vi "test-discretization.vi"(8 "error in (no error)":errorcluster) -> (0 "error out":errorcluster, 3 "All Tests Passed":bool)   [LabVIEW 2019]
uses:
  <vilib>/Analysis/Matrix/Datatypes/RealMatrix.ctl
  <vilib>/Analysis/baseanly.llb/Real A x B.vi
  <vilib>/Rock Robotics/WPI/ThirdParty/JAS_Junk/TrajLib/MatBuilder_Create.vi
  <vilib>/Rock Robotics/WPI/ThirdParty/JAS_Junk/TrajLib/MatrixHelper_CoerceSize.vi
  <vilib>/Rock Robotics/WPI/ThirdParty/JAS_Junk/TrajLib/Matrix_Exp.vi
  <vilib>/Rock Robotics/WPI/ThirdParty/JAS_Junk/TrajLib/Matrix_AssignBlock.vi
  <vilib>/Rock Robotics/WPI/ThirdParty/JAS_Junk/TrajLib/Matrix_ExtractFrom.vi
  <vilib>/Analysis/7linalg.llb/Transpose Matrix.vi
  <vilib>/Analysis/7linalg.llb/Real Transpose Matrix.vi
  <vilib>/Rock Robotics/WPI/ThirdParty/JAS_Junk/TrajLib/Matrix_Ident.vi
  <vilib>/Analysis/7linalg.llb/Matrix Exp.vi
  <vilib>/Analysis/7linalg.llb/Real Matrix Exp.vi
  <vilib>/Analysis/Matrix/Numeric/Multiply/Multiply.vi
  <vilib>/Analysis/Matrix/Numeric/Multiply/Multiply - RM,R.vi
  <vilib>/Analysis/7linalg.llb/Create Special Matrix.vi
  <vilib>/Analysis/7linalg.llb/Create Special Real Matrix.vi
  <vilib>/Analysis/Matrix/Numeric/Add/Add - RM,RM.vi
  <vilib>/Analysis/Matrix/Comparison/Equal/Equal - RM,RM.vi
  <vilib>/Rock Robotics/WPI/ThirdParty/JAS_Junk/TrajLib/Trajectory_Library.lvlib
  <vilib>/Analysis/NI_AALBase.lvlib
  <vilib>/Analysis/Matrix/NI_Matrix.lvlib
panel:
  out "X1Discrete 11":T1
  out "DiscB  11":T1
  out "Passed 11":bool
  out "DiscA  11":T1
  out "Passed 10":bool
  out "DiscA  10":T1
  out "Passed 16":bool
  out "DiscR  16":T1
  out "A+B Should be":T1
  out "A + B":T1
  out "Test x passed":bool
  out "Test 3 passed":bool
  out "Test Passed 2":bool
  out "Test Passed 1":bool
  out "Test Passed 0":bool
  out "AQ Passed":bool
  out "AQ - DiscQ":T1
  out "AQ - DiscA":T1
  out "AB-Taylor-Passed":bool
  out "ABTaylor-DiscB":T1
  out "ABTaylor - DiscA":T1
  out "AB-passed":bool
  out "AB-DiscB":T1
  out "AB - DiscA":T1
  out "x1-Disc":T1
  out "DiscA Error":bool
  out "DiscA":T1
  out "Cost Mat":T1
  out "CoVar Mat":T1
  # "1.0,   0.0,    0.0\n\n0.0,     4.0,   0.0, ;\n\n0.0,     0.0,  9.0;"
  # "1.0,      0.0,      0.0, \n\n0.0,   1.0 / 4.0,   0.0, \n\n0.0,       0.0,      1.0 / 9.0,"
  # "VecBuilder.fill(\n          x0.get(0, 0) + 1.0 * x0.get(1, 0), \n          x0.get(1, 0));"
  # "2,\n1"
  # "x0.get(0, 0) + x0.get(1, 0) + 0.5 * u.get(0, 0), \n\nx0.get(0, 0) + u.get(0, 0))"
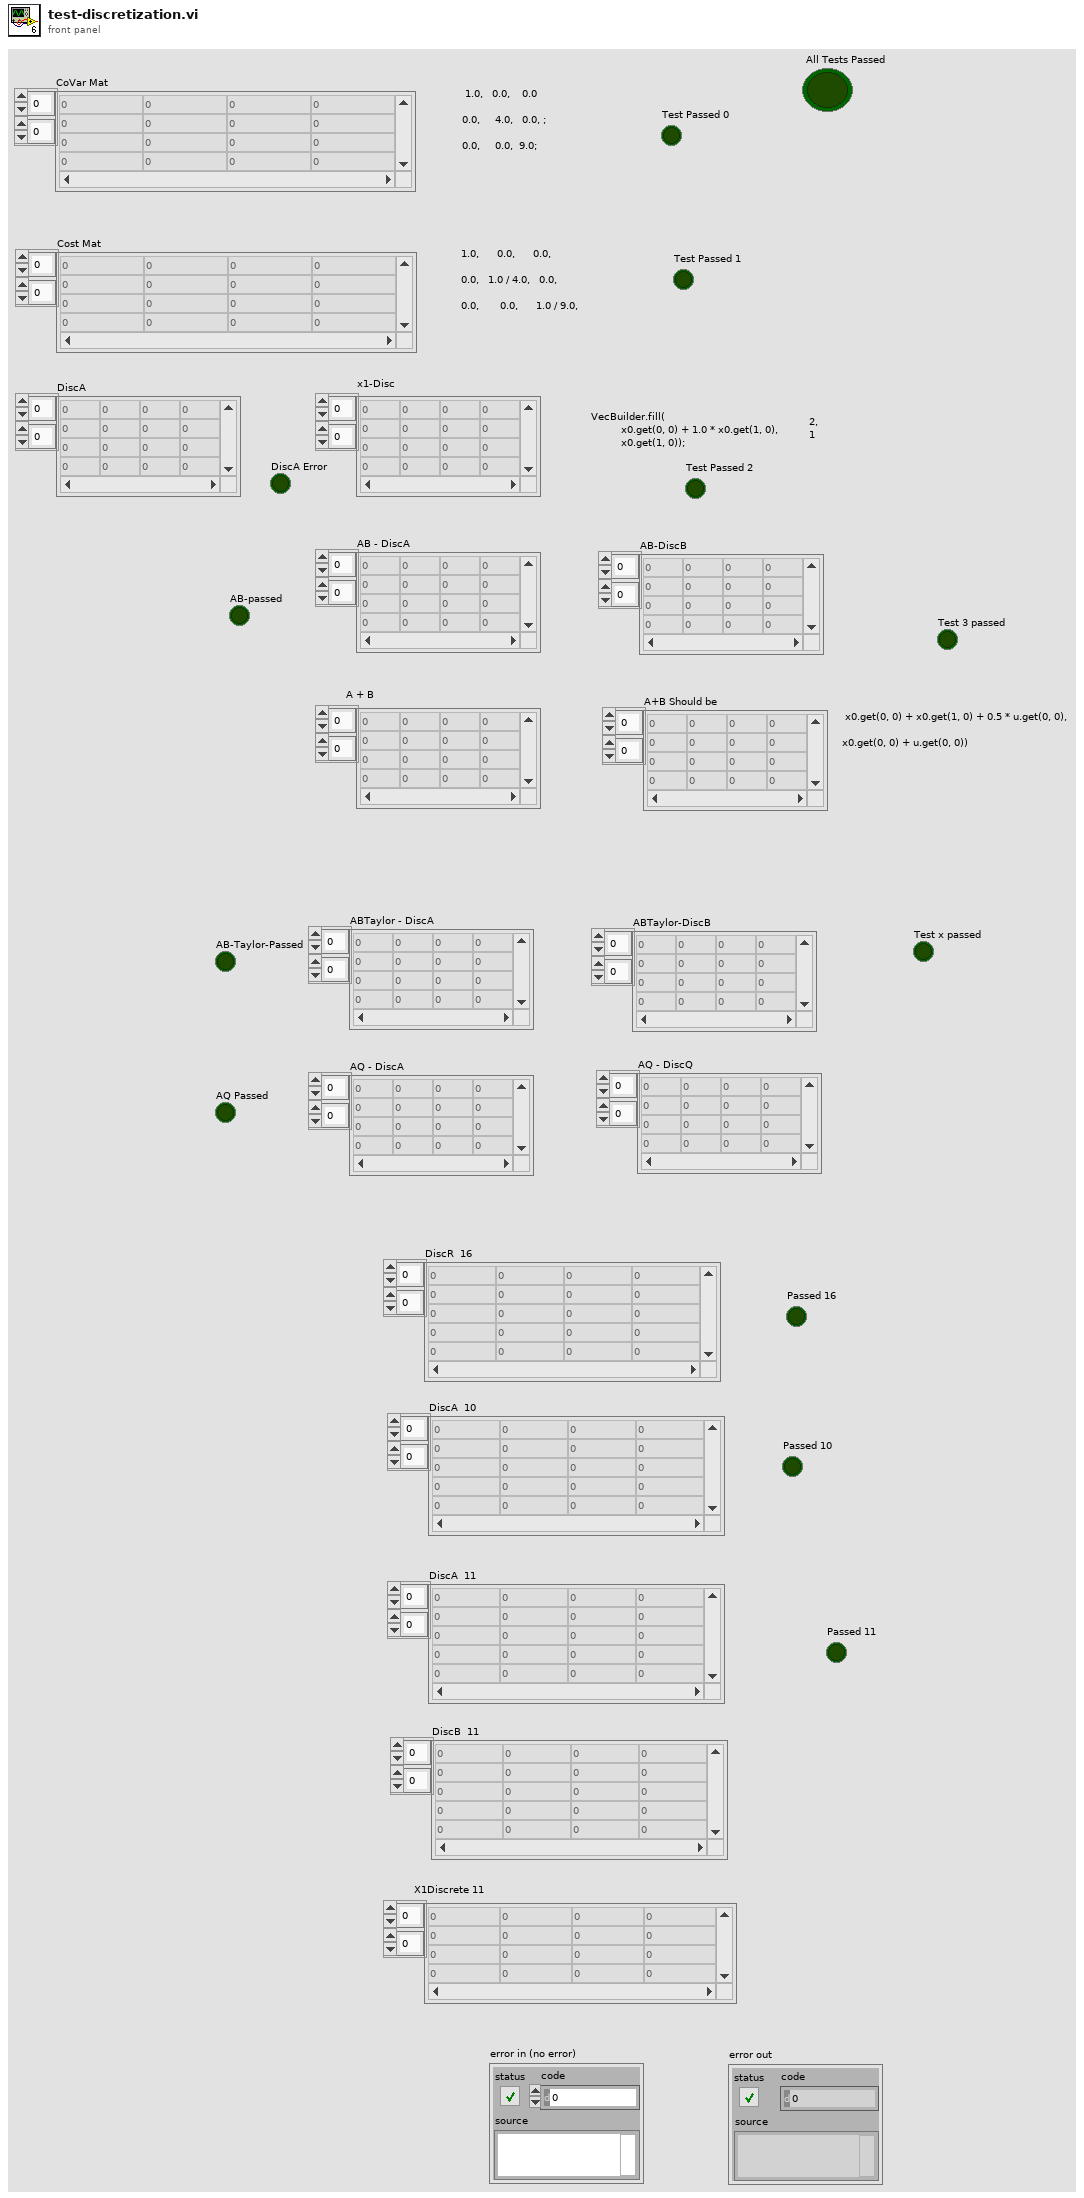
[diagram p1: front panel]
types:
  T1 = typedef "NI_Matrix.lvlib/RealMatrix.ctl" = dbl[][]
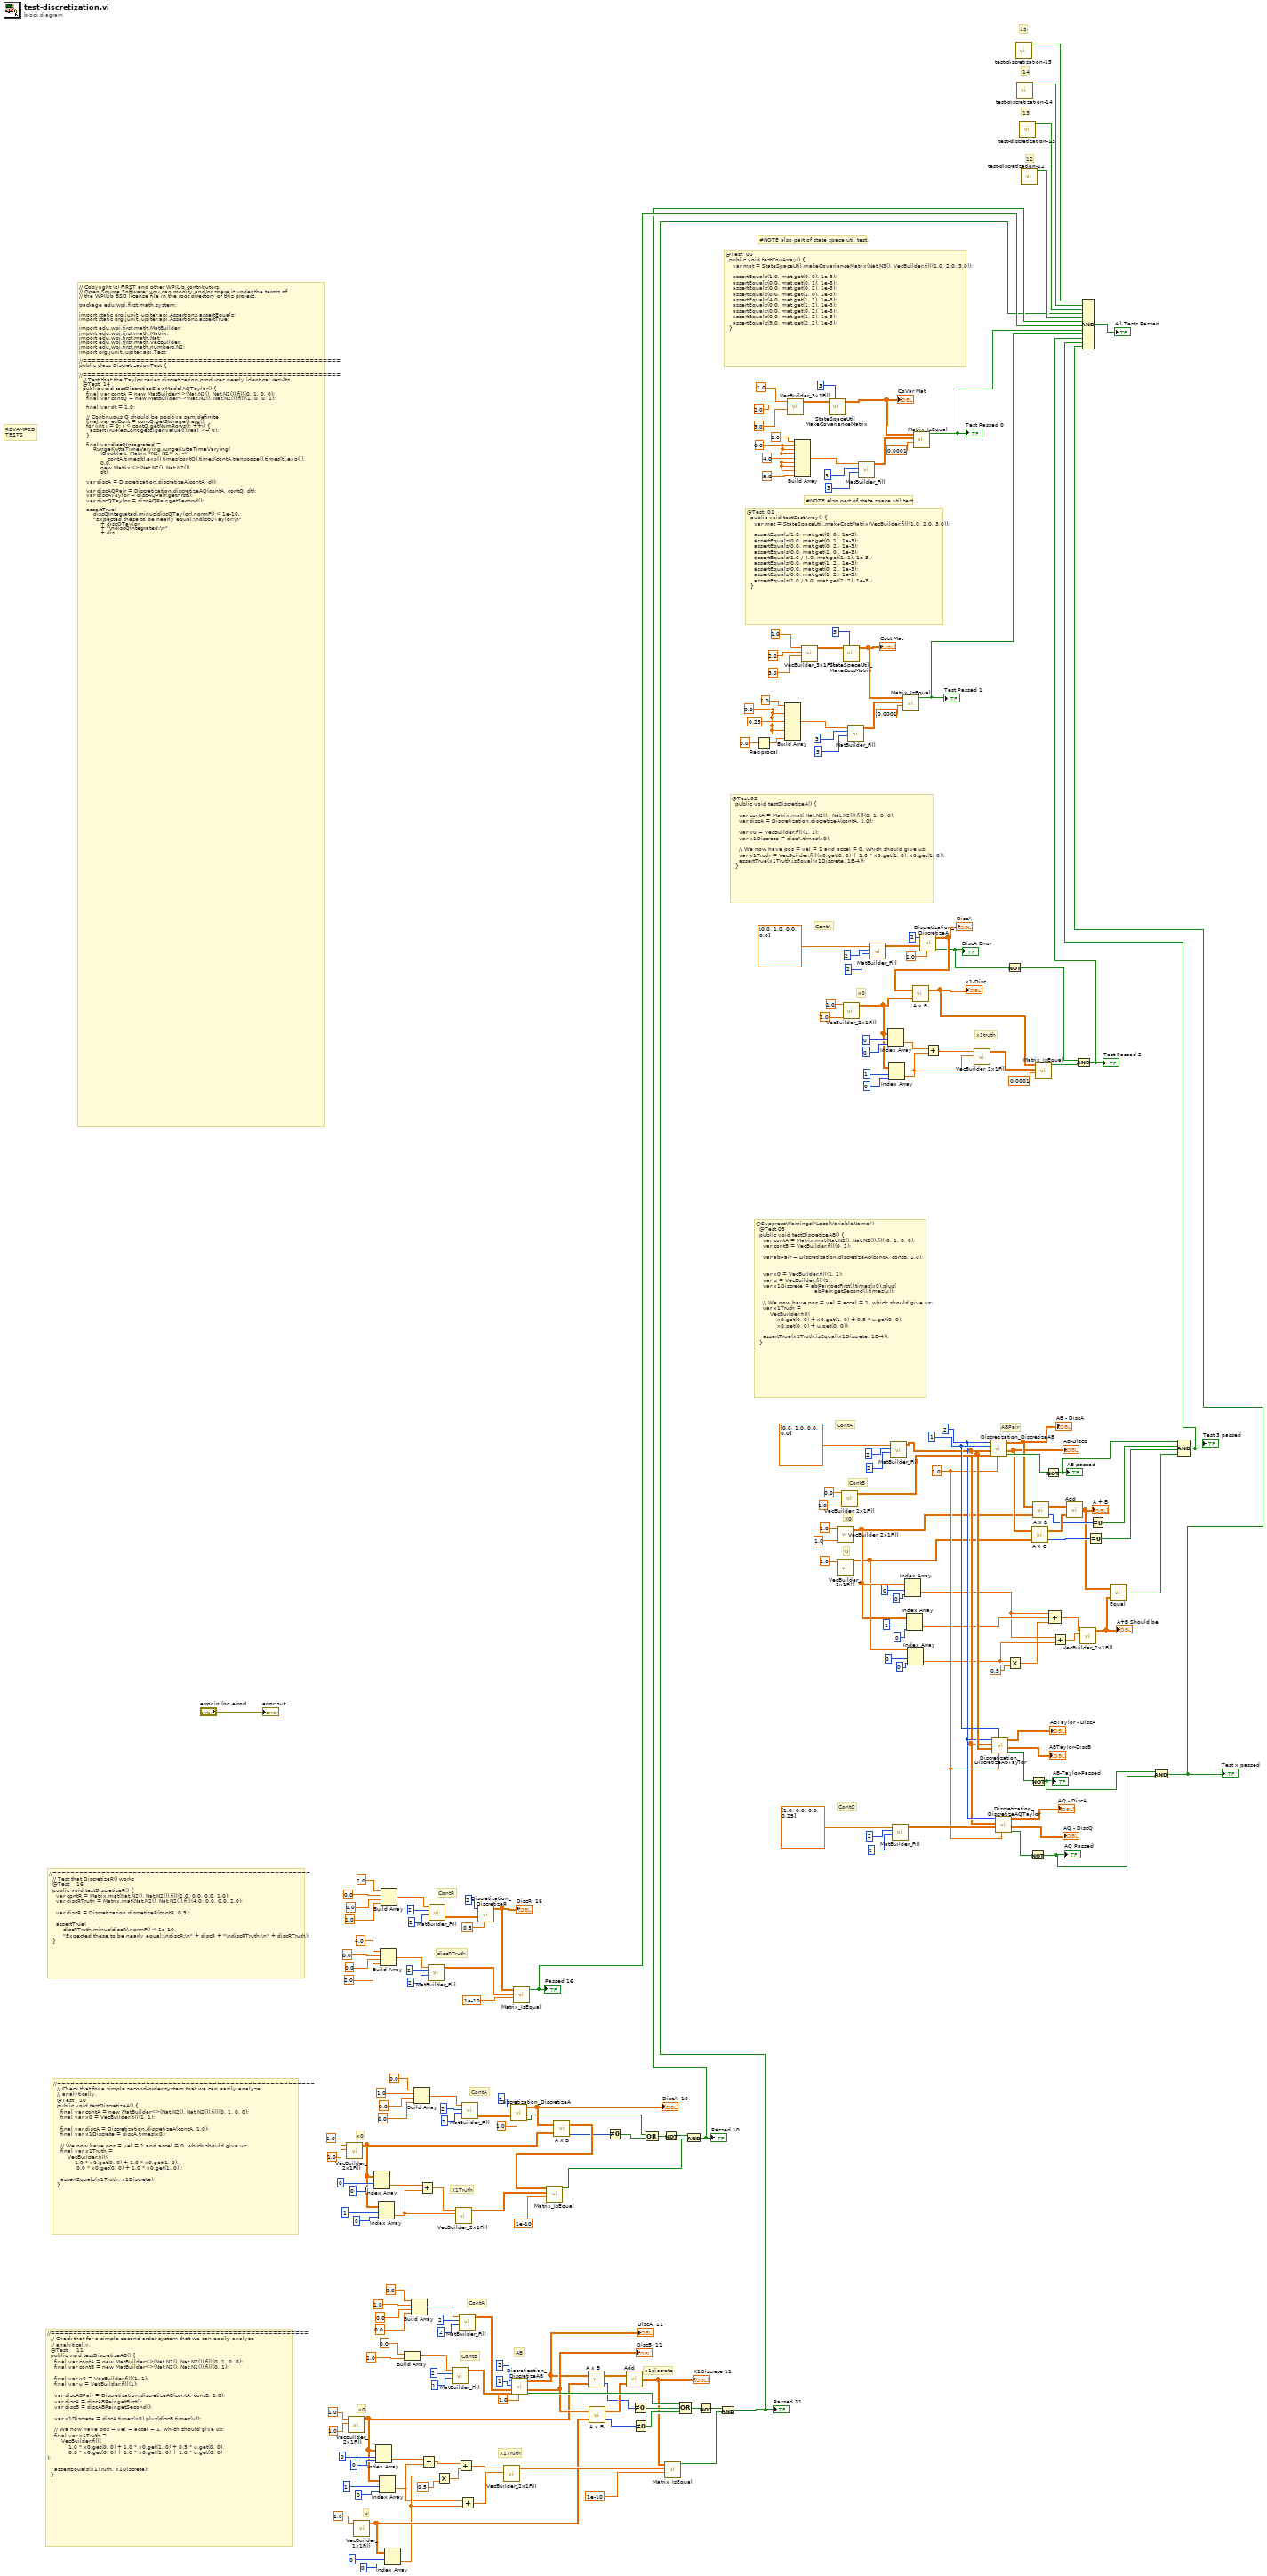
[diagram p0: block diagram]
diagram:
  w170 = 0.0 ("element")
  w180 = 0.0 ("element")
  w188 = 1.0 ("dT_Seconds")
  w198 = 1 ("Inputs")
  w191 = 2 ("States")
  # "#NOTE also part of state space util test."
  # "#NOTE also part of state space util test."
  # "15"
  # "14"
  # "13"
  # "AB"
  # "12"
  # "x1discrete"
  # "u"
  # "ContB"
  # "X1Truth"
  # "x0"
  # "ContA"
  # "//==========================================================\n  // Check that for a simple second-order system that we can easily analyze\n  // analytically,\n  @Test     11\n  public void testDiscretizeAB() {\n    final var contA = new MatBuilder<>(Nat.N2(), Nat.N2()).fill(0, 1, 0, 0);\n    final var contB = new MatBuilder<>(Nat.N2(), Nat.N1()).fill(0, 1);\n\n    final var x0 = VecBuilder.fill(1, 1);\n    final var u = VecBuilder.fill(1);\n\n    var discABPair = Discretization.discretizeAB(contA, contB, 1.0);\n    var discA = discABPair.getFirst();\n    var discB = discABPair.getSecond();\n\n    var x1Discrete = discA.times(x0).plus(discB.times(u));\n\n    // We now have pos = vel = accel = 1, which should give us:\n    final var x1Truth =\n        VecBuilder.fill(\n            1.0 * x0.get(0, 0) + 1.0 * x0.get(1, 0) + 0.5 * u.get(0, 0),\n            0.0 * x0.get(0, 0) + 1.0 * x0.get(1, 0) + 1.0 * u.get(0, 0)\n);\n\n    assertEquals(x1Truth, x1Discrete);\n  }"
  # "X1Truth"
  # "x0"
  # "ContA"
  # "//==========================================================\n  // Check that for a simple second-order system that we can easily analyze\n  // analytically,\n  @Test   10\n  public void testDiscretizeA() {\n    final var contA = new MatBuilder<>(Nat.N2(), Nat.N2()).fill(0, 1, 0, 0);\n    final var x0 = VecBuilder.fill(1, 1);\n\n    final var discA = Discretization.discretizeA(contA, 1.0);\n    final var x1Discrete = discA.times(x0);\n\n    // We now have pos = vel = 1 and accel = 0, which should give us:\n    final var x1Truth =\n        VecBuilder.fill(\n            1.0 * x0.get(0, 0) + 1.0 * x0.get(1, 0), \n             0.0 * x0.get(0, 0) + 1.0 * x0.get(1, 0));\n\n    assertEquals(x1Truth, x1Discrete);\n  }"
  # "discRTruth"
  # "ContR"
  # "//==========================================================\n  // Test that DiscretizeR() works\n  @Test    16\n  public void testDiscretizeR() {\n    var contR = Matrix.mat(Nat.N2(), Nat.N2()).fill(2.0, 0.0, 0.0, 1.0);\n    var discRTruth = Matrix.mat(Nat.N2(), Nat.N2()).fill(4.0, 0.0, 0.0, 2.0);\n\n    var discR = Discretization.discretizeR(contR, 0.5);\n\n    assertTrue(\n        discRTruth.minus(discR).normF() < 1e-10,\n        \"Expected these to be nearly equal:\\ndiscR:\\n\" + discR + \"\\ndiscRTruth:\\n\" + discRTruth);\n  }"
  # "REVAMPED\nTESTS"
  # "// Copyright (c) FIRST and other WPILib contributors.\n// Open Source Software; you can modify and/or share it under the terms of\n// the WPILib BSD license file in the root directory of this project.\n\npackage edu.wpi.first.math.system;\n\nimport static org.junit.jupiter.api.Assertions.assertEquals;\nimport static org.junit.jupiter.api.Assertions.assertTrue;\n\nimport edu.wpi.first.math.MatBuilder;\nimport edu.wpi.first.math.Matrix;\nimport edu.wpi.first.math.Nat;\nimport edu.wpi.first.math.VecBuilder;\nimport edu.wpi.first.math.numbers.N2;\nimport org.junit.jupiter.api.Test;\n\n//==========================================================\npublic class DiscretizationTest {\n\n//==========================================================\n  // Test that the Taylor series discretization produces nearly identical results.\n  @Test  14\n  public void testDiscretizeSlowModelAQTaylor() {\n    final var contA = new MatBuilder<>(Nat.N2(), Nat.N2()).fill(0, 1, 0, 0);\n    final var contQ = new MatBuilder<>(Nat.N2(), Nat.N2()).fill(1, 0, 0, 1);\n\n    final var dt = 1.0;\n\n    // Continuous Q should be positive semidefinite\n    final var esCont = contQ.getStorage().eig();\n    for (int i = 0; i < contQ.getNumRows(); ++i) {\n      assertTrue(esCont.getEigenvalue(i).real >= 0);\n    }\n\n    final var discQIntegrated =\n        RungeKuttaTimeVarying.rungeKuttaTimeVarying(\n            (Double t, Matrix<N2, N2> x) ->\n                contA.times(t).exp().times(contQ).times(contA.transpose().times(t).exp()),\n            0.0,\n            new Matrix<>(Nat.N2(), Nat.N2()),\n            dt);\n\n    var discA = Discretization.discretizeA(contA, dt);\n\n    var discAQPair = Discretization.discretizeAQ(contA, contQ, dt);\n    var discATaylor = discAQPair.getFirst();\n    var discQTaylor = discAQPair.getSecond();\n\n    assertTrue(\n        discQIntegrated.minus(discQTaylor).normF() < 1e-10,\n        \"Expected these to be nearly equal:\\ndiscQTaylor:\\n\"\n            + discQTaylor\n            + \"\\ndiscQIntegrated:\\n\"\n            + discQIntegrated);\n    assertTrue(discA.minus(discATaylor).normF() < 1e-10);\n\n    // Discrete Q should be positive semidefinite\n    final var esDisc = discQTaylor.getStorage().eig();\n    for (int i = 0; i < discQTaylor.getNumRows(); ++i) {\n      assertTrue(esDisc.getEigenvalue(i).real >= 0);\n    }\n  }\n\n//==========================================================\n  // Test that the Taylor series discretization produces nearly identical results.\n  @Test  15\n  public void testDiscretizeFastModelAQTaylor() {\n    final var contA = new MatBuilder<>(Nat.N2(), Nat.N2()).fill(0, 1, 0, -1500);\n    final var contQ = new MatBuilder<>(Nat.N2(), Nat.N2()).fill(0.0025, 0, 0, 1);\n\n    final var dt = 0.005;\n\n    // Continuous Q should be positive semidefinite\n    final var esCont = contQ.getStorage().eig();\n    for (int i = 0; i < contQ.getNumRows(); ++i) {\n      assertTrue(esCont.getEigenvalue(i).real >= 0);\n    }\n\n    final var discQIntegrated =\n        RungeKuttaTimeVarying.rungeKuttaTimeVarying(\n            (Double t, Matrix<N2, N2> x) ->\n                contA.times(t).exp().times(contQ).times(contA.transpose().times(t).exp()),\n            0.0,\n            new Matrix<>(Nat.N2(), Nat.N2()),\n            dt);\n\n    var discA = Discretization.discretizeA(contA, dt);\n\n    var discAQPair = Discretization.discretizeAQ(contA, contQ, dt);\n    var discATaylor = discAQPair.getFirst();\n    var discQTaylor = discAQPair.getSecond();\n\n    assertTrue(\n        discQIntegrated.minus(discQTaylor).normF() < 1e-3,\n        \"Expected these to be nearly equal:\\ndiscQTaylor:\\n\"\n            + discQTaylor\n            + \"\\ndiscQIntegrated:\\n\"\n            + discQIntegrated);\n    assertTrue(discA.minus(discATaylor).normF() < 1e-10);\n\n    // Discrete Q should be positive semidefinite\n    final var esDisc = discQTaylor.getStorage().eig();\n    for (int i = 0; i < discQTaylor.getNumRows(); ++i) {\n      assertTrue(esDisc.getEigenvalue(i).real >= 0);\n    }\n  }\n\n}"
  # "U"
  # "X0"
  # "ContB"
  # "ABPair"
  # "x1truth"
  # "x0"
  # "ContQ"
  # "ContA"
  # "@SuppressWarnings(\"LocalVariableName\")\n  @Test 03\n  public void testDiscretizeAB() {\n    var contA = Matrix.mat(Nat.N2(), Nat.N2()).fill(0, 1, 0, 0);\n    var contB = VecBuilder.fill(0, 1);\n\n    var abPair = Discretization.discretizeAB(contA, contB, 1.0);\n\n\n    var x0 = VecBuilder.fill(1, 1);\n    var u = VecBuilder.fill(1);\n    var x1Discrete = abPair.getFirst().times(x0).plus(\n                                 abPair.getSecond().times(u));\n\n    // We now have pos = vel = accel = 1, which should give us:\n    var x1Truth =\n        VecBuilder.fill(\n            x0.get(0, 0) + x0.get(1, 0) + 0.5 * u.get(0, 0), \n            x0.get(0, 0) + u.get(0, 0));\n\n    assertTrue(x1Truth.isEqual(x1Discrete, 1E-4));\n  }"
  # "ContA"
  # "@Test 02\n  public void testDiscretizeA() {\n\n    var contA = Matrix.mat( Nat.N2(),  Nat.N2()).fill(0, 1, 0, 0);\n    var discA = Discretization.discretizeA(contA, 1.0);\n\n    var x0 = VecBuilder.fill(1, 1);\n    var x1Discrete = discA.times(x0);\n\n    // We now have pos = vel = 1 and accel = 0, which should give us:\n    var x1Truth = VecBuilder.fill(x0.get(0, 0) + 1.0 * x0.get(1, 0), x0.get(1, 0));\n    assertTrue(x1Truth.isEqual(x1Discrete, 1E-4));\n  }"
  # "@Test  01\n  public void testCostArray() {\n    var mat = StateSpaceUtil.makeCostMatrix(VecBuilder.fill(1.0, 2.0, 3.0));\n\n    assertEquals(1.0, mat.get(0, 0), 1e-3);\n    assertEquals(0.0, mat.get(0, 1), 1e-3);\n    assertEquals(0.0, mat.get(0, 2), 1e-3);\n    assertEquals(0.0, mat.get(1, 0), 1e-3);\n    assertEquals(1.0 / 4.0, mat.get(1, 1), 1e-3);\n    assertEquals(0.0, mat.get(1, 2), 1e-3);\n    assertEquals(0.0, mat.get(0, 2), 1e-3);\n    assertEquals(0.0, mat.get(1, 2), 1e-3);\n    assertEquals(1.0 / 9.0, mat.get(2, 2), 1e-3);\n  }"
  # "@Test  00\n  public void testCovArray() {\n    var mat = StateSpaceUtil.makeCovarianceMatrix(Nat.N3(), VecBuilder.fill(1.0, 2.0, 3.0));\n\n    assertEquals(1.0, mat.get(0, 0), 1e-3);\n    assertEquals(0.0, mat.get(0, 1), 1e-3);\n    assertEquals(0.0, mat.get(0, 2), 1e-3);\n    assertEquals(0.0, mat.get(1, 0), 1e-3);\n    assertEquals(4.0, mat.get(1, 1), 1e-3);\n    assertEquals(0.0, mat.get(1, 2), 1e-3);\n    assertEquals(0.0, mat.get(0, 2), 1e-3);\n    assertEquals(0.0, mat.get(1, 2), 1e-3);\n    assertEquals(9.0, mat.get(2, 2), 1e-3);\n  }"
  n1 = call <vilib>:"VecBuilder_2x1Fill.vi"("R1"=1.0, "R0"=1.0) -> ("output matrix"=w70:T1)  [unwired: 9 in]
  n2 = call <vilib>:"VecBuilder_2x1Fill.vi"("R1"=1.0, "R0"=1.0) -> ("output matrix"=w24:T1)  [unwired: 9 in]
  n3 = call <vilib>:"VecBuilder_1x1Fill.vi"("R0_C0"=1.0 ("R0")) -> ("output matrix"=w15:T1)  [unwired: 10 in]
  n4 = Index Array(array=w70, index (row)=0, index (col)=0) -> (element=w67:dbl)
  n5 = Index Array(array=w24, index (row)=0, index (col)=0) -> (element=w41:dbl)
  n6 = Index Array(array=w70, index (row)=1, index (col)=0) -> (element=w66:dbl)
  n7 = Index Array(array=w24, index (row)=1, index (col)=0) -> (element=w9:dbl)
  n8 = Build Array(4.0 ("element"), 0.0 ("element"), 0.0 ("element"), 2.0 ("element")) -> (w102:dbl[])
  n9 = Build Array(2.0 ("element"), 0.0 ("element"), 0.0 ("element"), 1.0 ("element")) -> (w109:dbl[])
  n10 = Index Array(array=w15, index (row)=0, index (col)=0) -> (element=w10:dbl)
  n11 = Build Array(0.0 ("element"), 1.0 ("element")) -> (w35:dbl[])
  n12 = Build Array(0.0 ("element"), 1.0 ("element"), 0.0 ("element"), 0.0 ("element")) -> (w58:dbl[])
  n13 = Build Array(0.0 ("element"), 1.0 ("element"), 0.0 ("element"), 0.0 ("element")) -> (w88:dbl[])
  n14 = Add(x=w67, y=w66) -> (x+y=w68:dbl)
  n15 = Add(x=w41, y=w9) -> (x+y=w12:dbl)
  n16 = call <vilib>:"MatBuilder_Fill.vi"("Columns"=2, "Rows"=2, "Value List"=w102) -> ("output matrix"=w91:T1)  [unwired: 8 in]
  n17 = call <vilib>:"MatBuilder_Fill.vi"("Columns"=2, "Rows"=2, "Value List"=w109) -> ("output matrix"=w94:T1)  [unwired: 8 in]
  n18 = Multiply(x=w10, y=0.5) -> (x*y=w13:dbl)
  n19 = call <vilib>:"MatBuilder_Fill.vi"("Columns"=1, "Rows"=2, "Value List"=w35) -> ("output matrix"=w29:T1)  [unwired: 8 in]
  n20 = call <vilib>:"VecBuilder_2x1Fill.vi"("R1"=w66, "R0"=w68) -> ("output matrix"=w69:T1)  [unwired: 9 in]
  n21 = Add(x=w12, y=w13) -> (x+y=w11:dbl)
  n22 = call <vilib>:"MatBuilder_Fill.vi"("Columns"=2, "Rows"=2, "Value List"=w58) -> ("output matrix"=w30:T1)  [unwired: 8 in]
  n23 = Add(x=w9, y=w10) -> (x+y=w8:dbl)
  n24 = call <vilib>:"MatBuilder_Fill.vi"("Columns"=2, "Rows"=2, "Value List"=w88) -> ("output matrix"=w80:T1)  [unwired: 8 in]
  n25 = call <vilib>:"Discretization_DiscretizeR.vi"("dT_Seconds"=0.5, "ContR"=w94, "Outputs"=2) -> ("DiscR"=w93:T1)  [unwired: 7 in, 1 out]
  "DiscR  16" <- w93
  n26 = call <vilib>:"VecBuilder_2x1Fill.vi"("R1"=w8, "R0"=w11) -> ("output matrix"=w42:T1)  [unwired: 9 in]
  n27 = call <vilib>:"Discretization_DiscretizeA.vi"("dT_Seconds"=1.0, "ContA"=w80, "States"=2 ("Outputs")) -> ("Error"=w63:bool, "DiscA"=w75:T1)  [unwired: 7 in]
  "DiscA  10" <- w75
  n28 = call <vilib>:"Discretization_DiscretizeAB.vi"("dT_Seconds"=1.0, "ContB"=w29, "ContA"=w30, "Inputs"=1, "States"=2 ("Outputs")) -> ("Error"=w40:bool, "DiscB"=w26:T1, "DiscA"=w25:T1)  [unwired: 4 in]
  "DiscA  11" <- w25
  "DiscB  11" <- w26
  n29 = call <vilib>:"Matrix_IsEqual.vi"("Tolerance"=1e-10, "other"=w91, "input matrix"=w93) -> ("Equal"=w89:bool)  [unwired: 8 in]
  "Passed 16" <- w89
  n30 = call-poly <vilib>:"A x B.vi"("B"=w70, "A"=w75) -> ("error"=w64:i32, "A x B"=w65:T1)
  n31 = call <vilib>:"Matrix_IsEqual.vi"("Tolerance"=1e-10, "other"=w69, "input matrix"=w65) -> ("Equal"=w59:bool)  [unwired: 8 in]
  n32 = call-poly <vilib>:"A x B.vi"("B"=w24, "A"=w25) -> ("error"=w20:i32, "A x B"=w23:T1)
  n33 = call-poly <vilib>:"A x B.vi"("B"=w15, "A"=w26) -> ("error"=w19:i32, "A x B"=w22:T1)
  n34 = Not Equal To 0?(x=w64) -> (x != 0?=w62:bool)
  n35 = call-poly <vilib>:"Add.vi"("Real Matrix B"=w22, "Real Matrix A"=w23) -> ("A + B"=w18:T1)
  "X1Discrete 11" <- w18
  n36 = Not Equal To 0?(x=w20) -> (x != 0?=w39:bool)
  n37 = Not Equal To 0?(x=w19) -> (x != 0?=w21:bool)
  n38 = Compound Arithmetic op=OR(w63, w62) -> (w61:bool)
  n39 = Not(x=w61) -> (.not. x?=w60:bool)
  n40 = call <vilib>:"Matrix_IsEqual.vi"("Tolerance"=1e-10, "other"=w42, "input matrix"=w18) -> ("Equal"=w36:bool)  [unwired: 8 in]
  n41 = Compound Arithmetic op=OR(w40, w39, w21) -> (w38:bool)
  n42 = And(x=w60, y=w59) -> (x .and. y?=w7:bool)
  "Passed 10" <- w7
  n43 = Not(x=w38) -> (.not. x?=w37:bool)
  n44 = And(x=w37, y=w36) -> (x .and. y?=w4:bool)
  "Passed 11" <- w4
  n45 = Reciprocal(x=9.0 ("element")) -> (1/x=w166:dbl)
  n46 = Build Array(1.0 ("element"), w170, w170, w170, 0.25 ("element"), w170, w170, w170, w166) -> (w173:dbl[])
  n47 = call <vilib>:"VecBuilder_3x1Fill.vi"("R2"=3.0, "R1"=2.0, "R0"=1.0) -> ("output matrix"=w219:T1)  [unwired: 8 in]
  n48 = Build Array(1.0 ("element"), w180, w180, w180, 4.0 ("element"), w180, w180, w180, 9.0 ("element")) -> (w183:dbl[])
  n49 = call <vilib>:"VecBuilder_3x1Fill.vi"("R2"=3.0, "R1"=2.0, "R0"=1.0) -> ("output matrix"=w214:T1)  [unwired: 8 in]
  n50 = call <vilib>:"StateSpaceUtil_MakeCovarianceMatrix.vi"("States"=3, "StdDevs"=w219) -> ("Covariance Matrix"=w178:T1)  [unwired: 8 in, 1 out]
  "CoVar Mat" <- w178
  n51 = call <vilib>:"VecBuilder_2x1Fill.vi"("R1"=1.0, "R0"=1.0 ("R0_C0")) -> ("output matrix"=w121:T1)  [unwired: 9 in]
  n52 = call <vilib>:"VecBuilder_1x1Fill.vi"("R0_C0"=1.0) -> ("output matrix"=w120:T1)  [unwired: 10 in]
  n53 = call <vilib>:"VecBuilder_2x1Fill.vi"("R1"=1.0, "R0"=0.0 ("R0_C0")) -> ("output matrix"=w197:T1)  [unwired: 9 in]
  n54 = call <vilib>:"StateSpaceUtil_MakeCostMatrix.vi"("States"=3, "Costs"=w214) -> ("Costs Matrix"=w165:T1)  [unwired: 8 in, 1 out]
  "Cost Mat" <- w165
  n55 = call <vilib>:"VecBuilder_2x1Fill.vi"("R1"=1.0, "R0"=1.0 ("R0_C0")) -> ("output matrix"=w159:T1)  [unwired: 9 in]
  n56 = call <vilib>:"MatBuilder_Fill.vi"("Columns"=3, "Rows"=3, "Value List"=w173) -> ("output matrix"=w169:T1)  [unwired: 8 in]
  n57 = call <vilib>:"MatBuilder_Fill.vi"("Columns"=3, "Rows"=3, "Value List"=w183) -> ("output matrix"=w177:T1)  [unwired: 8 in]
  n58 = call <vilib>:"MatBuilder_Fill.vi"("Columns"=2, "Rows"=2, "Value List"=dbl[] [0.0, 1.0, 0.0, 0.0]) -> ("output matrix"=w207:T1)  [unwired: 8 in]
  n59 = Index Array(array=w159, index (row)=0, index (col)=0) -> (element=w158:dbl)
  n60 = Index Array(array=w159, index (row)=1, index (col)=0) -> (element=w156:dbl)
  n61 = call <vilib>:"MatBuilder_Fill.vi"("Columns"=2, "Rows"=2, "Value List"=dbl[] [0.0, 1.0, 0.0, 0.0]) -> ("output matrix"=w190:T1)  [unwired: 8 in]
  n62 = call <vilib>:"MatBuilder_Fill.vi"("Columns"=2, "Rows"=2, "Value List"=dbl[] [1.0, 0.0, 0.0, 0.25]) -> ("output matrix"=w189:T1)  [unwired: 8 in]
  n63 = call <vilib>:"Matrix_IsEqual.vi"("Tolerance"=0.0001, "other"=w169, "input matrix"=w165) -> ("Equal"=w149:bool)  [unwired: 8 in]
  "Test Passed 1" <- w149
  n64 = Index Array(array=w121, index (row)=0, index (col)=0) -> (element=w114:dbl)
  n65 = Index Array(array=w121, index (row)=1, index (col)=0) -> (element=w118:dbl)
  n66 = Index Array(array=w120, index (row)=0, index (col)=0) -> (element=w113:dbl)
  n67 = call <vilib>:"Matrix_IsEqual.vi"("Tolerance"=0.0001, "other"=w177, "input matrix"=w178) -> ("Equal"=w150:bool)  [unwired: 8 in]
  "Test Passed 0" <- w150
  n68 = call <vilib>:"Discretization_DiscretizeA.vi"("dT_Seconds"=1.0, "ContA"=w207, "States"=2) -> ("Error"=w152:bool, "DiscA"=w204:T1)  [unwired: 7 in]
  "DiscA" <- w204
  "DiscA Error" <- w152
  n69 = call-poly <vilib>:"A x B.vi"("B"=w159, "A"=w204) -> ("A x B"=w155:T1)  [unwired: 1 out]
  "x1-Disc" <- w155
  n70 = Add(x=w158, y=w156) -> (x+y=w157:dbl)
  n71 = call <vilib>:"VecBuilder_2x1Fill.vi"("R1"=w156, "R0"=w157) -> ("output matrix"=w154:T1)  [unwired: 9 in]
  n72 = call <vilib>:"Discretization_DiscretizeAB.vi"("dT_Seconds"=w188, "ContB"=w197, "ContA"=w190, "Inputs"=w198, "States"=w191) -> ("Error"=w146:bool, "DiscB"=w136:T1, "DiscA"=w140:T1)  [unwired: 4 in]
  "AB - DiscA" <- w140
  "AB-DiscB" <- w136
  n73 = call <vilib>:"Discretization_DiscretizeABTaylor.vi"("dT_Seconds"=w188, "Inputs"=w198, "ContB"=w197, "ContA"=w190, "States"=w191) -> ("Error"=w145:bool, "DiscB"=→"ABTaylor-DiscB":T1, "DiscA"=→"ABTaylor - DiscA":T1)  [unwired: 4 in]
  n74 = call <vilib>:"Discretization_DiscretizeAQTaylor.vi"("dT_Seconds"=w188, "ContQ"=w189, "ContA"=w190, "States"=w191) -> ("Error"=w143:bool, "DiscQ"=→"AQ - DiscQ":T1, "DiscA"=→"AQ - DiscA":T1)  [unwired: 5 in]
  n75 = Not(x=w152) -> (.not. x?=w151:bool)
  n76 = Multiply(x=w113, y=0.5) -> (x*y=w117:dbl)
  n77 = call "test-discretization-15.vi"() -> ("All Tests Passed"=w1:bool)  [unwired: 10 in, 1 out]
  n78 = call "test-discretization-14.vi"() -> ("All Tests Passed"=w2:bool)  [unwired: 10 in, 1 out]
  n79 = call "test-discretization-13.vi"() -> ("All Tests Passed"=w3:bool)  [unwired: 10 in, 1 out]
  n80 = call "test-discretization-12.vi"() -> ("All Tests Passed"=w5:bool)  [unwired: 10 in, 1 out]
  n81 = Not(x=w143) -> (.not. x?=w141:bool)
  "AQ Passed" <- w141
  n82 = Not(x=w145) -> (.not. x?=w142:bool)
  "AB-Taylor-Passed" <- w142
  n83 = call-poly <vilib>:"A x B.vi"("B"=w120, "A"=w136) -> ("error"=w132:i32, "A x B"=w134:T1)
  n84 = call-poly <vilib>:"A x B.vi"("B"=w121, "A"=w140) -> ("error"=w133:i32, "A x B"=w135:T1)
  n85 = call <vilib>:"Matrix_IsEqual.vi"("Tolerance"=0.0001, "other"=w154, "input matrix"=w155) -> ("Equal"=w153:bool)  [unwired: 8 in]
  n86 = Not(x=w146) -> (.not. x?=w144:bool)
  "AB-passed" <- w144
  n87 = Compound Arithmetic op=ADD(w114, w118, w117) -> (w116:dbl)
  n88 = Add(x=w114, y=w113) -> (x+y=w115:dbl)
  n89 = call-poly <vilib>:"Add.vi"("Real Matrix B"=w134, "Real Matrix A"=w135) -> ("A + B"=w111:T1)
  "A + B" <- w111
  n90 = Compound Arithmetic op=AND(w151, w153) -> (w148:bool)
  "Test Passed 2" <- w148
  n91 = call <vilib>:"VecBuilder_2x1Fill.vi"("R1"=w115, "R0"=w116) -> ("output matrix"=w112:T1)  [unwired: 9 in]
  "A+B Should be" <- w112
  n92 = Equal To 0?(x=w132) -> (x = 0?=w130:bool)
  n93 = Equal To 0?(x=w133) -> (x = 0?=w131:bool)
  n94 = call-poly <vilib>:"Equal.vi"("Real Matrix B"=w112, "Real Matrix A"=w111) -> ("A = B?"=w110:bool)
  n95 = Compound Arithmetic op=AND(w142, w141) -> (w128:bool)
  "Test x passed" <- w128
  n96 = Compound Arithmetic op=AND(w144, w131, w130, w110) -> (w129:bool)
  "Test 3 passed" <- w129
  n97 = Compound Arithmetic op=AND(w1, w2, w3, w4, w5, w7, w89, w150, w149, w148, w129, w128) -> (→"All Tests Passed":bool)
  "error out" <- "error in (no error)"
